vi "ReadTDMSTest1.vi"() -> ()   [LabVIEW 2016]
panel:
  out "property value":string
  in  "file path":path
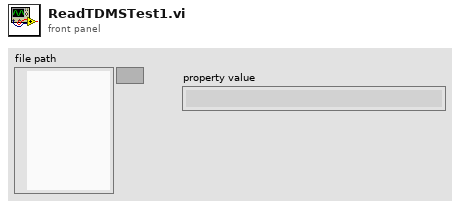
[diagram p1: front panel]
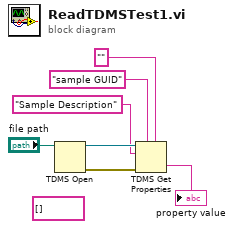
[diagram p0: block diagram]
diagram:
  (unwired) string[] [] ("data")
  n1 = TDMS Open(11:"file path") -> (0:w6:errorcluster, 3:w5:refnum<k34>)  [unwired: 6 in]
  n2 = TDMS Get Properties(5:"" ("name"), 7:"sample GUID" ("name"), 8:w6, 10:"Sample Description" ("group name in"), 11:w5) -> (4:→"property value":string)  [unwired: 1 in, 5 out]
